vi "Find Inherited VIs.vi"(8 "error in (no error)":errorcluster, 11 "LVClassLibrary in":refnum<vi>) -> (0 "error out":errorcluster, 2 "Inherited Dynamic Member VIs":refnum<vi>[](array[refnum]))   [LabVIEW 2020, in "LUnit Test Case.lvclass"]
uses:
  LUnit Test Case/LUnit Test Case.lvclass
  LUnit Test Case/LUnit Test Case.lvclass/LUnit Test Case.ctl
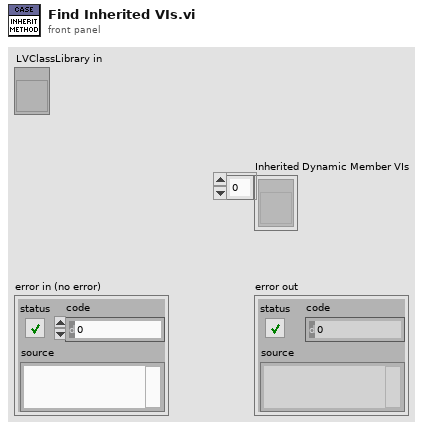
[diagram p1: front panel]
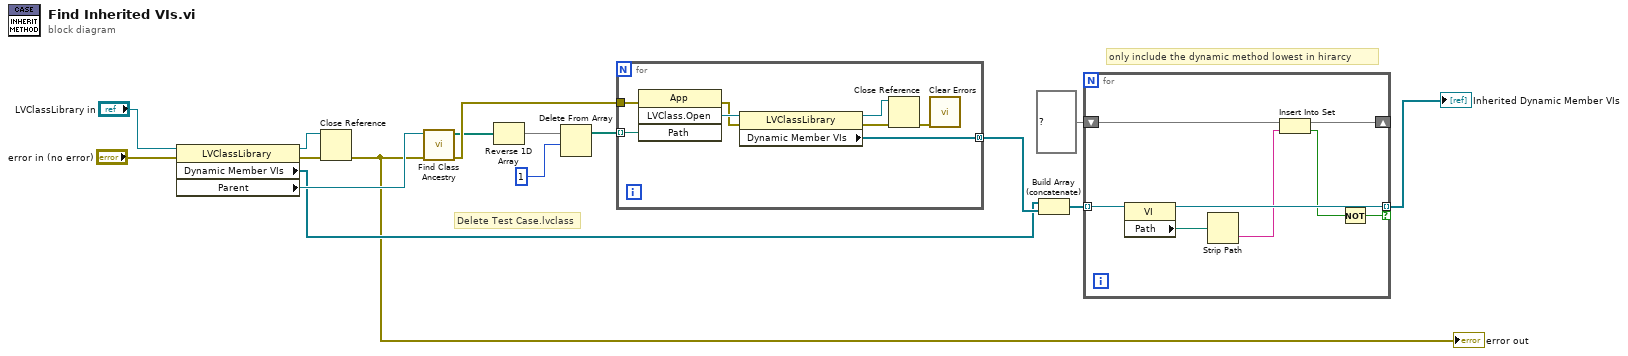
[diagram p0: block diagram]
diagram:
  # "Delete Test Case.lvclass"
  # "only include the dynamic method lowest in hirarcy"
  n1 = property class="LVClassLibrary"(reference="LVClassLibrary in", error in="error in (no error)") -> (reference out=w1:refnum<vi>, error out=w6:errorcluster, "Dynamic Member VIs"=w3:refnum<vi>[], "Parent"=w5:refnum<vi>)
  n2 = Close Reference(reference=w1, error in (no error)=w6) -> (error out=w2:errorcluster)
  "error out" <- w2
  n3 = call "Find Class Ancestry.vi"("error in (no error)"=w2, "reference in"=w5) -> ("error out"=w12:errorcluster, "Class Ancestry"=w11:path[])  [unwired: 8 in]
  n4 = Reverse 1D Array(array=w11) -> (reversed array=w10:path[])
  n5 = Delete From Array(array=w10, length=1) -> (array with subset deleted=w13:path[])  [unwired: 1 in, 1 out]
  n6 = for {
    tunnel: w13 -> [w24] mode=indexing
    tunnel: [w22] -> w16 mode=concatenating
    tunnel: w12 -> [w17]
    n7 = invoke class="App" method="LVClass.Open"(error in=w17, "Path"=w24) -> (error out=w20:errorcluster, "LVClass.Open"=w23:refnum<vi>)  [unwired: 2 in, 2 out]
    n8 = property class="LVClassLibrary"(reference=w23, error in=w20) -> (reference out=w18:refnum<vi>, error out=w19:errorcluster, "Dynamic Member VIs"=w22:refnum<vi>[])
    n9 = Close Reference(reference=w18, error in (no error)=w19) -> (error out=w21:errorcluster)
    n10 = call <vilib>:"Clear Errors.vi"("error in (no error)"=w21) -> ()  [unwired: 5 in, 2 out]
  }
  n11 = Build Array (concatenate)(w3, w16) -> (w4:refnum<vi>[])
  n12 = for {
    tunnel: [w31] -> w15 mode=indexing if=w25
    tunnel: w4 -> [w32] mode=indexing
    shift-right: [w28] -> _
    shift-left: set{string} {} ("set") -> [w29]
    n13 = property class="VI"(reference=w32) -> (reference out=w31:refnum<vi>, "Path"=w30:path)  [unwired: 1 in, 1 out]
    n14 = Strip Path(path=w30) -> (name=w27:string)  [unwired: 1 out]
    n15 = Insert Into Set(10:w27, 11:w29) -> (2:w26:bool, 3:w28:set{string})
    n16 = Not(x=w26) -> (.not. x?=w25:bool)
  }
  "Inherited Dynamic Member VIs" <- w15
